vi "Add Remote Terminal.vi"(8 "error in":errorcluster, 9 "terminal name":string, 10 "terminal address":T1, 11 "port":T2 format="%.0x") -> (0 "error out":errorcluster, 2 "remote terminal":T2 format="%.0x", 3 "port out":T2 format="%.0x")   [LabVIEW 2020, in "AIM MIL-STD-1553 Scripting.lvlib"]
doc: "Adds a remote terminal with <b>terminal address</b> to the <b>port</b> and returns the newly added <b>remote terminal</b> reference. Also adds a Status Channel and the Start/Stop Command Channels to the Remote Terminal, unless it has a terminal address of 31 (reserved for broadcast option)."
uses:
  AIM MIL-STD-1553 Scripting.lvlib
  <vilib>/NI VeriStand/Custom Device API/Custom Device Item Ref.ctl
  Shared/Address.ctl
  Constants.vi
  <vilib>/NI VeriStand/Custom Device API/Custom Device API.lvlib
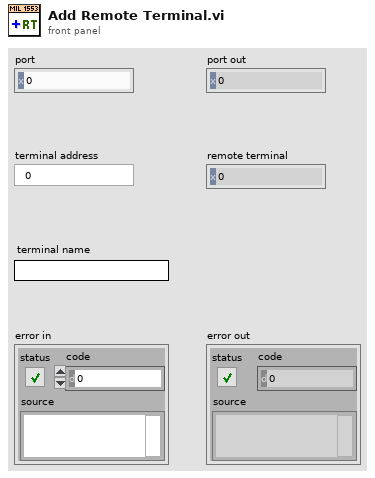
[diagram p1: front panel]
types:
  T1 = typedef "Address.ctl" = u16
  T2 = typedef "Custom Device API.lvlib/Custom Device Item Ref.ctl" = u64
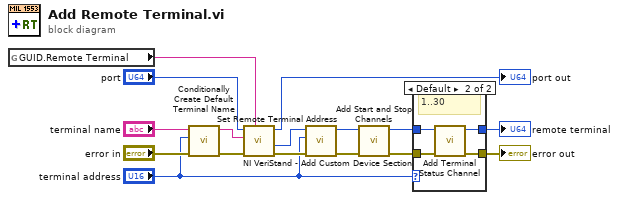
[diagram p0: block diagram]
diagram:
  n1 = global read "Constants.vi" "GUID.Remote Terminal"() -> (w16:string)
  n2 = call "Conditionally Create Default Terminal Name.vi"("error in"="error in", "terminal address"="terminal address", "terminal name"="terminal name") -> ("error out"=w12:errorcluster, "terminal name out"=w6:string)  [unwired: 7 in]
  n3 = call <vilib>:"NI VeriStand - Add Custom Device Section.vi"("GUID (Default Section)"=w16, "error in (no error)"=w12, "Section Name"=w6, "Parent Ref in"="port") -> ("error out"=w5:errorcluster, "Section Ptr"=w2:T2, "Parent Ref out"=→"port out":T2)  [unwired: 4 in, 1 out]
  n4 = call "Set Remote Terminal Address.vi"("error in"=w5, "terminal address"="terminal address", "remote terminal"=w2) -> ("error out"=w3:errorcluster, "remote terminal out"=w4:T2)  [unwired: 7 in]
  n5 = call "Add Start and Stop Channels.vi"("error in"=w3, "terminal"=w4) -> ("error out"=w10:errorcluster, "terminal out"=w9:T2)  [unwired: 6 in, 2 out]
  n6 = case shown="Default" "terminal address" {
    tunnel: [w18 w22] -> w11
    tunnel: w10 -> [w18 w21]
    tunnel: w9 -> [w17 w20]
    tunnel: [w17 w19] -> w8
    frame 31 {
      # "Broadcast"
    }
    frame Default {
      # "1..30"
      n7 = call "Add Terminal Status Channel.vi"("error in"=w21, "terminal"=w20) -> ("error out"=w22:errorcluster, "terminal out"=w19:T2)  [unwired: 7 in, 1 out]
    }
  }
  "error out" <- w11
  "remote terminal" <- w8
